vi "string2refnum.vi"(7 "String":string, 10 "Control in":refnum<vi>) -> ()   [LabVIEW 2013]
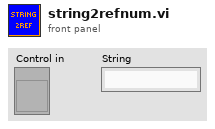
[diagram p1: front panel]
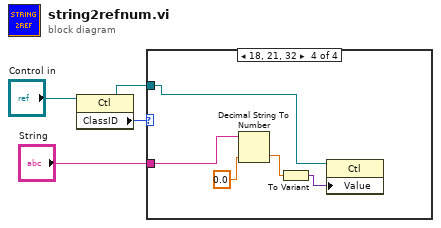
[diagram p0: block diagram]
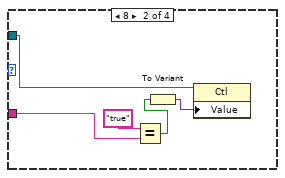
[diagram p3: hidden frame]
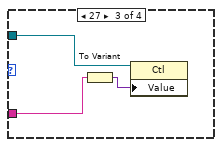
[diagram p4: hidden frame]
diagram:
  n1 = property class="Ctl"(reference="Control in") -> ("ClassID"=w3:u32)  [unwired: 1 in, 2 out]
  n2 = case shown="18, 21, 32" w3 {
    tunnel: "String" -> [_ w8 w10 w15]
    tunnel: "Control in" -> [_ w4 w9 w12]
    frame Default {
      # "Unknown class id\nleave ref value unchanged"
    }
    frame 8 {
      n3 = Equal?(x="true", y=w8) -> (x = y?=w6:bool)
      n4 = To Variant(anything=w6) -> (Variant=w5:variant)
      n5 = property class="Ctl"(reference=w4, "Value"=w5) -> ()  [unwired: 1 in, 2 out]
    }
    frame 27 {
      n6 = To Variant(anything=w10) -> (Variant=w11:variant)
      n7 = property class="Ctl"(reference=w9, "Value"=w11) -> ()  [unwired: 1 in, 2 out]
    }
    frame 18, 21, 32 {
      n8 = Decimal String To Number(string=w15, default (0L)=0.0) -> (number=w13:dbl)  [unwired: 1 in, 1 out]
      n9 = To Variant(anything=w13) -> (Variant=w16:variant)
      n10 = property class="Ctl"(reference=w12, "Value"=w16) -> ()  [unwired: 1 in, 2 out]
    }
  }
